vi "Read Reply.vi"(8 "error in (no error)":errorcluster, 11 "GenericCommClass in":refnum<class "ASCIICommClass.lvclass">) -> (0 "error out":errorcluster, 2 "Reply":string, 3 "GenericCommClass out":refnum<class "ASCIICommClass.lvclass">)   [LabVIEW 2013, in "ASCIICommClass.lvclass"]
uses:
  ASCIICommClass.lvclass
  ASCIICommClass.lvclass/ASCIICommClass.ctl
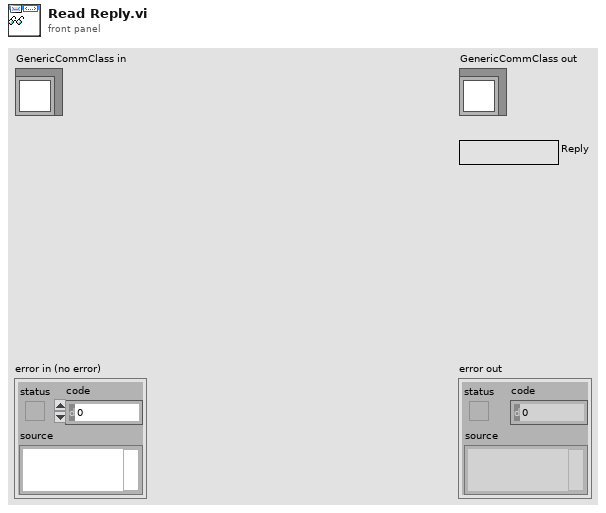
[diagram p1: front panel]
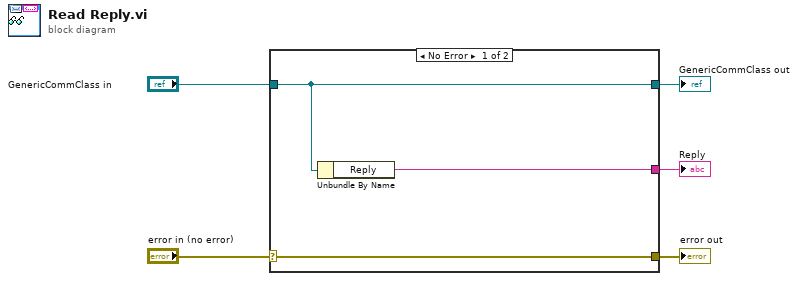
[diagram p0: block diagram]
diagram:
  n1 = case shown="No Error" "error in (no error)" {
    selector: "error in (no error)" -> [w8 w9]
    tunnel: [w8 w9] -> w4
    tunnel: [w7 w10] -> w2
    tunnel: "GenericCommClass in" -> [w7 w10]
    tunnel: [w6 _] -> w1
    frame No Error {
      n2 = Unbundle By Name(w7) -> ("Reply"=w6:string)
    }
    frame Error {
    }
  }
  "error out" <- w4
  "GenericCommClass out" <- w2
  "Reply" <- w1
